vi "Configure Protocol Settings.vi"(8 "error in":errorcluster, 11 "Protocol settings":T1={"Protocol capture resource name"="", "Data line"=0, "Channel"=0, "Clock rate"=12288000, "Number of words"=19200, "Sensitivity"=0.34762, "Frame sync edge for channel 0"=enum."Falling", "Channel count per frame"=2, "Channel length"=32, "Bit depth"=24, "Channel 0 offset"=1, "Endianness"=enum."MSB First", "Data justification"=enum."Left Justified", "Frame length"=64, "Frame sync pulse width"=32, "Bit clock edge sync"=enum."Falling"}) -> (0 "error out":errorcluster, 3 "PDM task":T2)   [LabVIEW 2021, in "audio adc shared.lvlib"]
uses:
  <vilib>/PDM Acquisition Toolkit/host/Classes/Tasks/PCM Input/Controls/DVR PCM Input Task.ctl
  <vilib>/PDM Acquisition Toolkit/host/Classes/Tasks/PCM Input/PCM Input Task.lvclass
  controls/Protocol Settings.ctl
  <vilib>/PDM Acquisition Toolkit/host/Classes/Tasks/PDM Tasks/Controls/Acquisition Mode.ctl
  <vilib>/PDM Acquisition Toolkit/host/Classes/Session/Controls/Logic Levels.ctl
  <vilib>/PDM Acquisition Toolkit/shared/controls/PCM Data Format Configuration.ctl
  <vilib>/PDM Acquisition Toolkit/shared/controls/Digital Edge.ctl
  <vilib>/PDM Acquisition Toolkit/shared/controls/PCM Bit Endianness.ctl
  <vilib>/PDM Acquisition Toolkit/shared/controls/PCM Data Justification.ctl
  <vilib>/PDM Acquisition Toolkit/shared/controls/PCM Frame Sync Control.ctl
  <vilib>/PDM Acquisition Toolkit/host/API/Public/Create Tasks/Create PCM Input Task.vi
  <vilib>/PDM Acquisition Toolkit/host/API/Public/Configure/Timing/Configure Timing - PCM Input Slave.vi
  <vilib>/PDM Acquisition Toolkit/host/API/Public/Configure/PDM Channel/Configure Microphone Sensitivity FSPA - PCM Input Task.vi
  audio adc shared.lvlib
  <vilib>/PDM Acquisition Toolkit/host/Classes/Session/DecoderSession.lvclass
  <vilib>/PDM Acquisition Toolkit/host/API/PDM Acquisition Toolkit.lvlib
  <vilib>/PDM Acquisition Toolkit/shared/PDM Shared.lvlib
  <vilib>/PDM Acquisition Toolkit/host/Classes/Tasks/PDM Tasks/PDM Task.lvclass
  controls/audio adc controls.lvlib
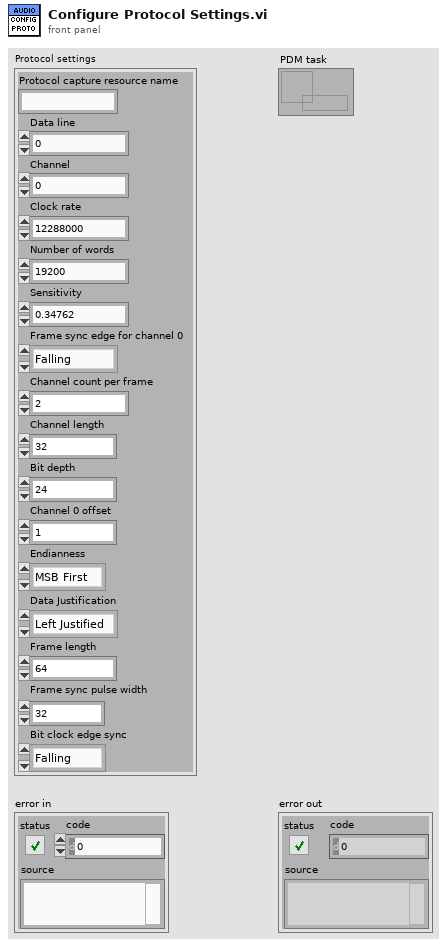
[diagram p1: front panel]
types:
  T1 = typedef "audio adc controls.lvlib/Protocol Settings.ctl" = cluster{"Protocol capture resource name":string, "Data line":u16, "Channel":u32, "Clock rate":u32, "Number of words":i32, "Sensitivity":dbl, "Frame sync edge for channel 0":enum32{"Rising", "Falling"}, "Channel count per frame":u8, "Channel length":u16, "Bit depth":u8, "Channel 0 offset":u16, "Endianness":enum32{"MSB First", "LSB First"}, "Data justification":enum32{"Left Justified", "Right Justified"}, "Frame length":u16, "Frame sync pulse width":u16, "Bit clock edge sync":enum32{"Rising", "Falling"}}
  T2 = typedef "PDM Acquisition Class Library.lvlib/PCM Input Task.lvclass/DVR PCM Input Task.ctl" = refnum<data-value>
  T3 = typedef "PDM Shared.lvlib/PCM Frame Sync Control.ctl" = cluster{"Frame Length":u16, "Frame Sync Pulse Width":u16, "Bit Clock Edge  Sync":T4}
  T4 = typedef "PDM Shared.lvlib/Digital Edge.ctl" = enum8{"Rising", "Falling"}
  T5 = typedef "PDM Shared.lvlib/PCM Data Format Configuration.ctl" = cluster{"Frame Sync Edge for Channel 0":T4, "Channel Count Per Frame":u8, "Channel Length":u16, "Bit Depth":u8, "Channel 0 Offset":u16, "Endianness":T6, "Data Justification":T7}
  T6 = typedef "PDM Shared.lvlib/PCM Bit Endianness.ctl" = enum16{"MSB First", "LSB First"}
  T7 = typedef "PDM Shared.lvlib/PCM Data Justification.ctl" = enum16{"Left Justified", "Right Justified"}
  T8 = typedef "PDM Acquisition Class Library.lvlib/DecoderSession.lvclass/Logic Levels.ctl" = enum16{"3.3 V", "1.8 V", "1.2 V"}
  T9 = typedef "PDM Acquisition Class Library.lvlib/PDM Task.lvclass/Acquisition Mode.ctl" = enum16{"Finite", "Continuous"}
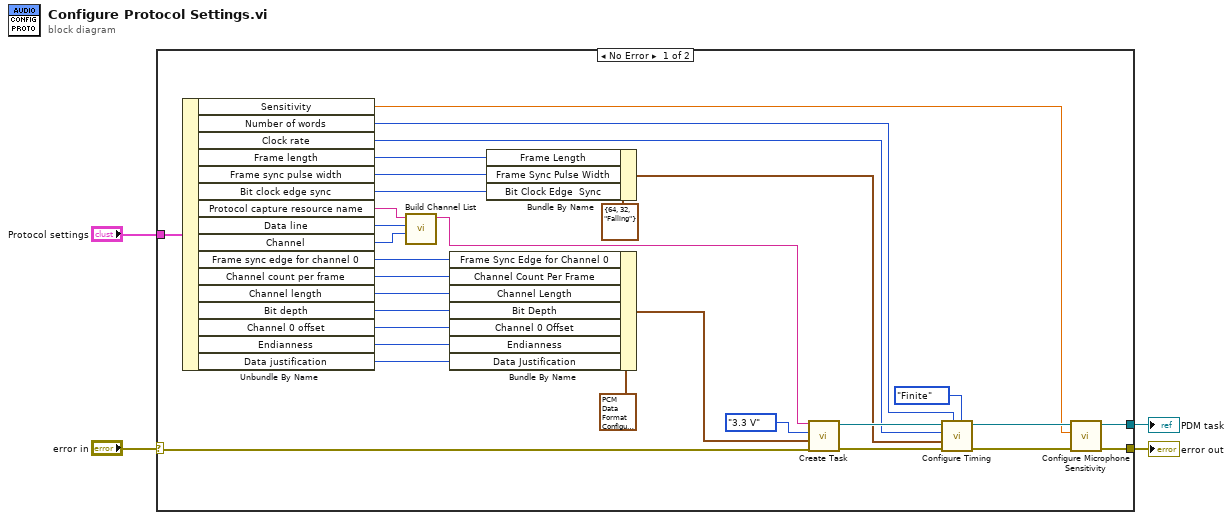
[diagram p0: block diagram]
diagram:
  n1 = case shown="No Error" "error in" {
    selector: "error in" -> [w28 w36]
    tunnel: [w22 w36] -> w2
    tunnel: [w31 _] -> w3
    tunnel: "Protocol settings" -> [w27 _]
    frame No Error {
      n2 = Unbundle By Name(w27) -> ("Sensitivity"=w5:dbl, "Number of words"=w30:i32, "Clock rate"=w29:u32, "Frame length"=w14:u16, "Frame sync pulse width"=w13:u16, "Bit clock edge sync"=w12:enum32{"Rising", "Falling"}, "Protocol capture resource name"=w9:string, "Data line"=w8:u16, "Channel"=w7:u32, "Frame sync edge for channel 0"=w17:enum32{"Rising", "Falling"}, "Channel count per frame"=w15:u8, "Channel length"=w16:u16, "Bit depth"=w21:u8, "Channel 0 offset"=w20:u16, "Endianness"=w19:enum32{"MSB First", "LSB First"}, "Data justification"=w18:enum32{"Left Justified", "Right Justified"})
      n3 = call "Build Channel List.vi"("Channel"=w7, "Data line"=w8, "Protocol capture resource name"=w9) -> ("String"=w6:string)  [unwired: 8 in]
      n4 = Bundle By Name(cluster=T5 {"Frame Sync Edge for Channel 0"=enum."Falling", "Channel Count Per Frame"=2, "Channel Length"=32, "Bit Depth"=24, "Channel 0 Offset"=1, "Endianness"=enum."MSB First", "Data Justification"=enum."Left Justified"} ("PCM data configuration"), "Frame Sync Edge for Channel 0"=w17, "Channel Count Per Frame"=w15, "Channel Length"=w16, "Bit Depth"=w21, "Channel 0 Offset"=w20, "Endianness"=w19, "Data Justification"=w18) -> (w25:T5)
      n5 = Bundle By Name(cluster=T3 {"Frame Length"=64, "Frame Sync Pulse Width"=32, "Bit Clock Edge  Sync"=enum."Falling"} ("Frame Sync Clock Control"), "Frame Length"=w14, "Frame Sync Pulse Width"=w13, "Bit Clock Edge  Sync"=w12) -> (w23:T3)
      n6 = call-poly <vilib>:"Create Task.vi"("error in"=w28, "PCM data configuration"=w25, "logic level"=Logic_Levels."3.3 V", "channel list"=w6) -> ("error out"=w34:errorcluster, "PCM input task out"=w35:T2)  [unwired: 6 in]
      n7 = call-poly <vilib>:"Configure Timing.vi"("acquisition mode"=Acquisition_Mode."Finite", "Frame Sync Clock Control"=w23, "number of words per channel"=w30, "error in"=w34, "Bit Clock rate"=w29, "PCM input task in"=w35) -> ("error out"=w10:errorcluster, "PCM input task out"=w11:T2)  [unwired: 4 in]
      n8 = call-poly <vilib>:"Configure Microphone Sensitivity.vi"("error in"=w10, "microphone sensitivity (FS/Pa)"=w5, "PCM input task in"=w11) -> ("error out"=w22:errorcluster, "PCM input task out"=w31:T2)  [unwired: 7 in]
    }
    frame Error {
    }
  }
  "PDM task" <- w3
  "error out" <- w2
